vi "Save Text Data.vi"(0 "String":string, 1 "Archive File Type":T1, 2 "LogFile Type":T2=enum."DLL  Errors", 3 "error in":errorcluster) -> (5 "New File":bool, 6 "error out":errorcluster)   [LabVIEW 2009]
uses:
  LogFileType.ctl
  Archive File Type.ctl
  Log Filename Actions.ctl
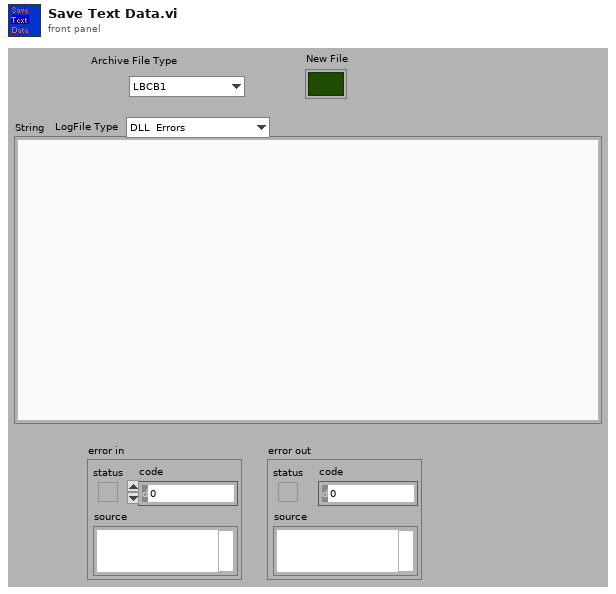
[diagram p1: front panel]
types:
  T1 = typedef "Archive File Type.ctl" = enum16{"LBCB1", "LBCB2", "ExternalSensors", "Combined"}
  T2 = typedef "LogFileType.ctl" = enum16{"Continuous", "Step", "Volts", "Offsets", "DLL  Errors", "Snapshot", "Commands", "StiffnessUpdates", "End List"}
  T3 = enum16{"open", "replace", "create", "open or create", "replace or create", "replace or create with confirmation"}
  T4 = typedef "Log Filename Actions.ctl" = enum16{"Init", "Get Filename", "New Log Directory"}
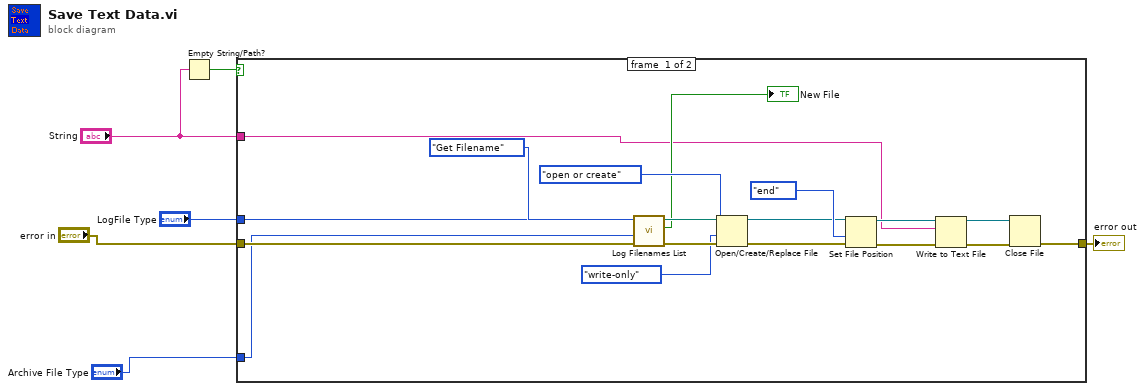
[diagram p0: block diagram]
diagram:
  n1 = Empty String/Path?(string/path="String") -> (empty?=w2:bool)
  n2 = case shown="False" w2 {
    tunnel: "error in" -> [w24 w25]
    tunnel: [w17 w25] -> w5
    tunnel: "LogFile Type" -> [w9 _]
    tunnel: "String" -> [w8 _]
    tunnel: "Archive File Type" -> [w7 _]
    frame #0 {
      n3 = call "Log Filenames List.vi"("error in (no error)"=w24, "Archive File Type"=w7, "LogFile Type"=w9, "Log Filename Actions"=Log_Filename_Actions."Get Filename") -> ("error out"=w16:errorcluster, "New File"=→"New File":bool, "Filename"=w12:path)  [unwired: 5 out]
      n4 = Open/Create/Replace File(file path (use dialog)=w12, error in=w16, operation (0:open)=T3."open or create", access (0:read/write)=enum16{"read/write", "read-only", "write-only"}."write-only") -> (refnum out=w19:refnum<file>, error out=w20:errorcluster)  [unwired: 3 out]
      n5 = Set File Position(refnum=w19, from (0:start)=enum16{"start", "end", "current"}."end", error in=w20) -> (refnum out=w22:refnum<file>, error out=w21:errorcluster)  [unwired: 1 out]
      n6 = Write to Text File(file (use dialog)=w22, text=w8, error in=w21) -> (refnum out=w15:refnum<file>, error out=w14:errorcluster)  [unwired: 2 out]
      n7 = Close File(refnum=w15, error in=w14) -> (error out=w17:errorcluster)  [unwired: 1 out]
    }
    frame #1 {
    }
  }
  "error out" <- w5
